vi "AddParamChannels.vi"(6 "Type":T3, 8 "error in":errorcluster, 9 "Initial Value":u32, 10 "Parameters to add":T2[](array[typedef]), 11 "Node Ref In":T1=18446744073709551615 format="%.0x") -> (0 "error out":errorcluster, 3 "Node Ref Out":T1=18446744073709551615 format="%.0x")   [LabVIEW 2011, in "AIT 429 Custom Device.lvlib"]
uses:
  AIT 429 Custom Device.lvlib
  <vilib>/NI Veristand/Custom Device API/Custom Device Item Ref.ctl
  <vilib>/NI Veristand/Custom Device API/Custom Device Channel Type.ctl
  Controls/ARINCParam.ctl
  <vilib>/NI Veristand/Custom Device API/Custom Device Channel.ctl
  Controls and Global/Global.vi
  <vilib>/NI Veristand/Custom Device API/Custom Device API.lvlib
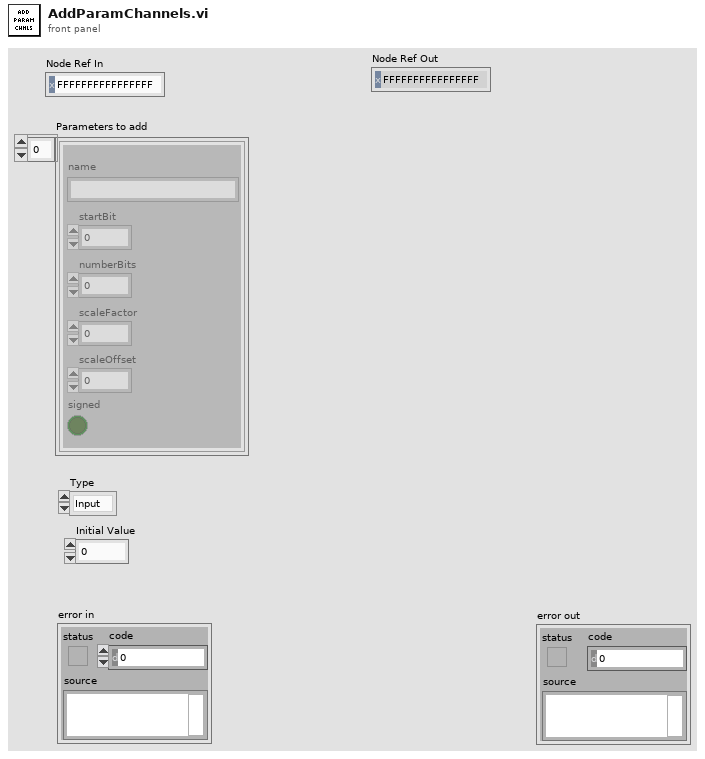
[diagram p1: front panel]
types:
  T1 = typedef "Custom Device API.lvlib/Custom Device Item Ref.ctl" = u64
  T2 = typedef "AIT 429 Custom Device.lvlib/ARINCParam.ctl" = cluster{"name":string, "startBit":i32, "numberBits":i32, "scaleFactor":dbl, "scaleOffset":dbl, "signed":bool}
  T3 = typedef "Custom Device API.lvlib/Custom Device Channel Type.ctl" = enum16{"Input", "Output"}
  T4 = typedef "Custom Device API.lvlib/Custom Device Channel.ctl" = cluster{"Type":T3, "Units":string, "Default Value":dbl, "Faultable":bool, "Scalable":bool}
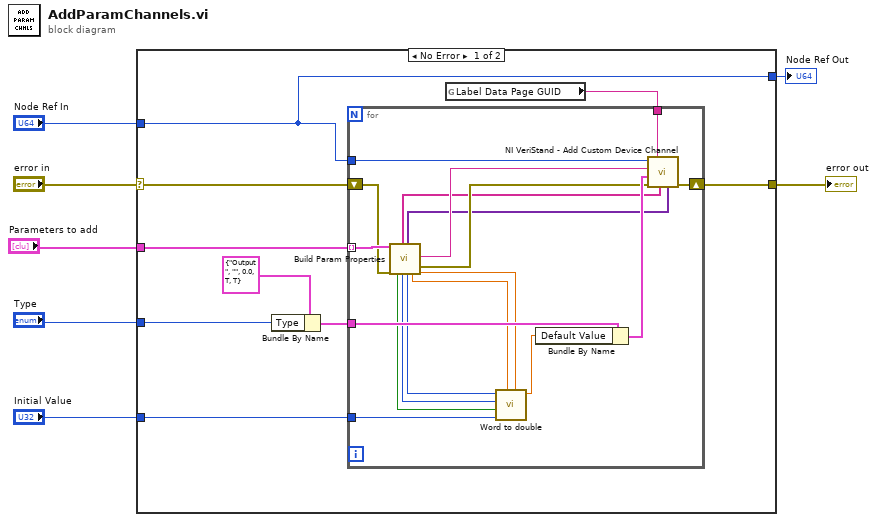
[diagram p0: block diagram]
diagram:
  n1 = case shown="No Error" "error in" {
    selector: "error in" -> [w9 w36]
    tunnel: "Parameters to add" -> [w13 _]
    tunnel: "Node Ref In" -> [w8 w35]
    tunnel: "Initial Value" -> [w12 _]
    tunnel: "Type" -> [w11 _]
    tunnel: [w10 w36] -> w4
    tunnel: [w8 w35] -> w1
    frame No Error {
      n2 = Bundle By Name(cluster=T4 {"Type"=enum."Output", "Units"="", "Default Value"=0.0, "Faultable"=TRUE, "Scalable"=TRUE} ("Channel"), "Type"=w11) -> (w15:T4)
      n3 = global read "Global.vi" "Label Data Page GUID"() -> (w16:string)
      n4 = for {
        shift-right: [w34] -> w10
        shift-left: w9 -> [w27]
        tunnel: w8 -> [w33]
        tunnel: w15 -> [w31]
        tunnel: w16 -> [w32]
        tunnel: w13 -> [w28] mode=indexing
        tunnel: w12 -> [w29]
        n5 = call "Build Param Properties.vi"("ARINC Parameter"=w28, "error in (no error)"=w27) -> ("signed"=w21:bool, "Prop Names"=w24:string[], "numberBits"=w20:i32, "Prop Values"=w23:variant[], "startBit"=w19:i32, "scaleFactor"=w18:dbl, "name"=w25:string, "error out"=w26:errorcluster, "scaleOffset"=w17:dbl)  [unwired: 9 in]
        n6 = call "Word to double.vi"("ScaleOffset (0)"=w17, "ScaleFac (1)"=w18, "word"=w29, "Signed? (F)"=w21, "Number of Bits"=w20, "Start Bit"=w19) -> ("Double"=w22:dbl)  [unwired: 5 in]
        n7 = Bundle By Name(cluster=w31, "Default Value"=w22) -> (w30:T4)
        n8 = call <vilib>:"NI VeriStand - Add Custom Device Channel.vi"("Property Values"=w23, "Property names"=w24, "GUID (Default Channel)"=w32, "error in (no error)"=w26, "Channel"=w30, "Channel Name"=w25, "Parent Ref in"=w33) -> ("error out"=w34:errorcluster)  [unwired: 1 in, 3 out]
      }
    }
    frame Error {
    }
  }
  "error out" <- w4
  "Node Ref Out" <- w1
